vi "face_eye_Detection_test_realTime.vi"() -> ()   [LabVIEW 2010]
uses:
  <vilib>/vision/driver/NI_Vision_Acquisition_Software.lvlib
  <libdir>/resource/objmgr/imaqdx.rc
  <vilib>/vision/NI_Vision_Development_Module.lvlib
  D:/1. DELO FAKS/MOJE/3. Moj OpenCV_dll/face_detection_haar_DLL/build/Release/face_detection_haar_DLL.dll
  <vilib>/Analysis/NI_AALBase.lvlib
  <vilib>/Analysis/baseanly.llb/Mean (DBL).vi
  <vilib>/userdefined/High Color/IMAQdx.ctl
panel:
  out "average detection time [ms]":dbl format="%0.2f"
  out "detected eyes":i32
  out "detected faces":i32
  in  "STOP":bool
  in  "camera":T1="cam0"
  out "processing \ntime [ms]":u32
  out "cascade classifiers loaded?":bool
  out "Image":T2(plugin-control)
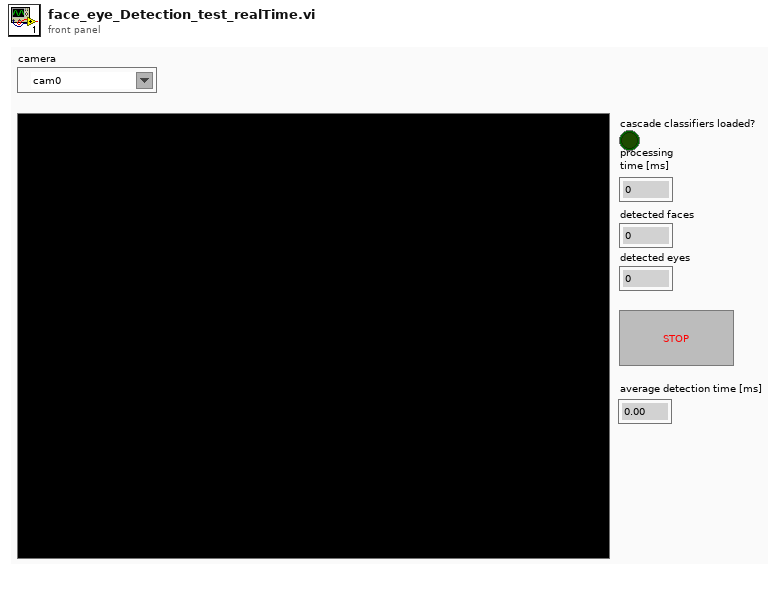
[diagram p1: front panel]
types:
  T1 = typedef "IMAQdx.ctl" = refnum<k21>
  T2 = typedef "IMAQ Image.ctl" = refnum<image>
  T3 = typedef "Image Type" = u32
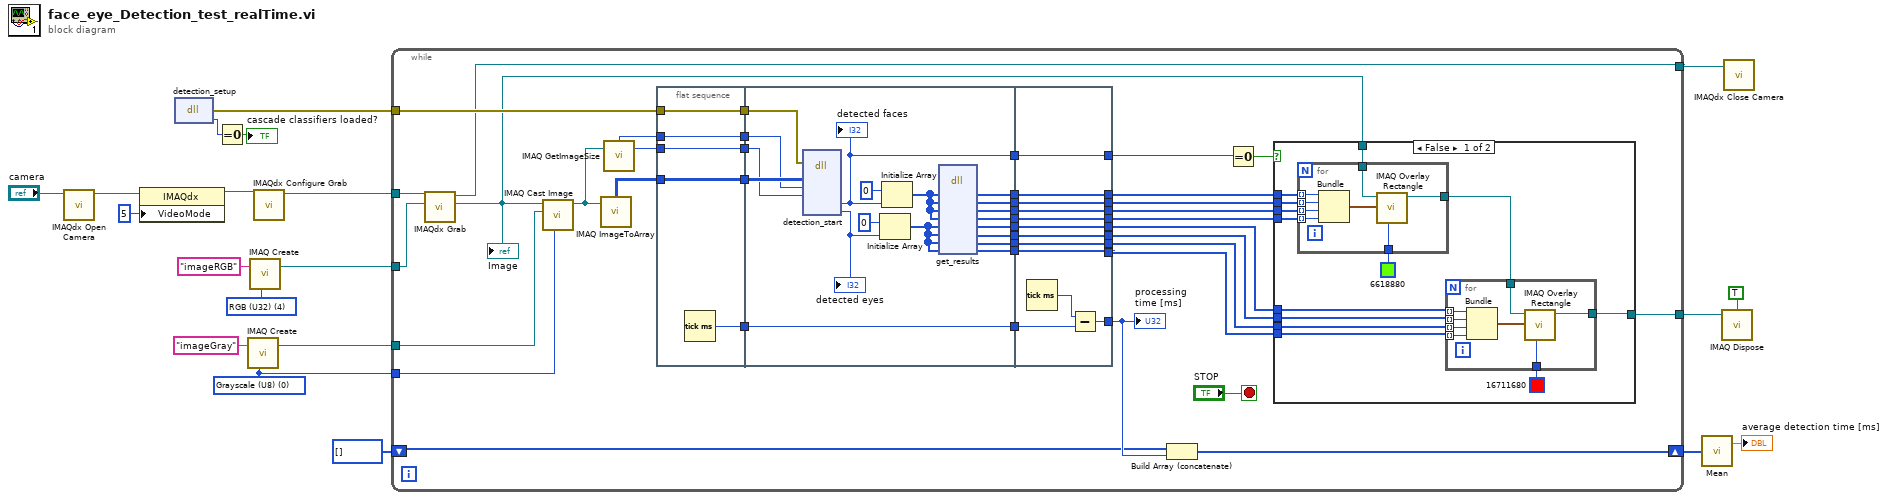
[diagram p0: block diagram]
diagram:
  w6 = T3 0 items=["Grayscale (U8)", "Grayscale (I16)", "Grayscale (SGL)", "Complex (CSG)", "RGB (U32)", "HSL (U32)", "RGB (U64)", "Grayscale (U16)"] ("Image Type")
  w19 = T3 4 items=["Grayscale (U8)", "Grayscale (I16)", "Grayscale (SGL)", "Complex (CSG)", "RGB (U32)", "HSL (U32)", "RGB (U64)", "Grayscale (U16)"] ("Image Type")
  n1 = call <vilib>:"IMAQdx Open Camera.vi"("Session In"="camera") -> ("Session Out"=w14:T1)  [unwired: 9 in, 1 out]
  n2 = property class="IMAQdx"(reference=w14, "VideoMode"=u32 5) -> (reference out=w13:T1)  [unwired: 1 in, 1 out]
  n3 = dll-call lib="D:/1. DELO FAKS/MOJE/3. Moj OpenCV_dll/face_detection_haar_DLL/build/Release/face_detection_haar_DLL.dll" fn="detection_setup"() -> (error out=w18:errorcluster, "return type"=w17:i32)  [unwired: 3 in, 1 out]
  n4 = Equal To 0?(x=w17) -> (x = 0?=→"cascade classifiers loaded?":bool)
  n5 = call "IMAQ Create"("Image Name"="imageGray", "Image Type"=w6) -> ("New Image"=w7:T2)  [unwired: 3 in, 1 out]
  n6 = call "IMAQ Create"("Image Name"="imageRGB", "Image Type"=w19) -> ("New Image"=w10:T2)  [unwired: 3 in, 1 out]
  n7 = call <vilib>:"IMAQdx Configure Grab.vi"("Session In"=w13) -> ("Session Out"=w11:T1)  [unwired: 9 in, 1 out]
  n8 = while {
    tunnel: w18 -> [w51]
    tunnel: w11 -> [w42]
    tunnel: w10 -> [w41]
    tunnel: [w40] -> w9
    tunnel: w7 -> [w38]
    tunnel: w6 -> [w37]
    tunnel: [w24] -> w4
    shift-right: [w22] -> w2
    shift-left: u32[] [] -> [w21]
    stop <- "STOP" stop-if-true
    n9 = call <vilib>:"IMAQdx Grab.vi"("Image In"=w41, "Session In"=w42) -> ("Image Out"=w35:T2, "Session Out"=w40:T1)  [unwired: 6 in, 2 out]
    "Image" <- w35
    n10 = call "IMAQ Cast Image"("Image Type"=w37, "Image Dst"=w38, "Image Src"=w35) -> ("Image Dst Out"=w39:T2)  [unwired: 7 in, 1 out]
    n11 = call "IMAQ ImageToArray"("Image"=w39) -> ("Image Pixels (U8)"=w46:u8[][])  [unwired: 3 in, 4 out]
    n12 = call "IMAQ GetImageSize"("Image"=w39) -> ("Y Resolution"=w44:i32, "X Resolution"=w45:i32)  [unwired: 3 in, 1 out]
    n13 = flat-sequence {
      tunnel: w51 -> [w96]
      tunnel: [w96] -> w61
      tunnel: [w95] -> w60
      tunnel: w46 -> [w94]
      tunnel: [w94] -> w59
      tunnel: w45 -> [w93]
      tunnel: [w93] -> w58
      tunnel: [w92] -> w57
      tunnel: w44 -> [w92]
      tunnel: w61 -> [w115]
      tunnel: [w112] -> w56
      tunnel: [w111] -> w55
      tunnel: [w110] -> w54
      tunnel: [w109] -> w53
      tunnel: [w108] -> w52
      tunnel: w60 -> [w108]
      tunnel: w59 -> [w107]
      tunnel: w58 -> [w106]
      tunnel: w57 -> [w105]
      tunnel: [w102] -> w34
      tunnel: [w101] -> w33
      tunnel: [w100] -> w32
      tunnel: [w99] -> w31
      tunnel: [w98] -> w30
      tunnel: [w124] -> w47
      tunnel: [w125] -> w48
      tunnel: [w126] -> w49
      tunnel: [w127] -> w50
      tunnel: w56 -> [w127]
      tunnel: w55 -> [w126]
      tunnel: w54 -> [w125]
      tunnel: w53 -> [w124]
      tunnel: w52 -> [w122]
      tunnel: [w121] -> w23
      tunnel: w34 -> [w120]
      tunnel: w33 -> [w119]
      tunnel: w32 -> [w118]
      tunnel: w31 -> [w117]
      tunnel: [w120] -> w28
      tunnel: [w119] -> w27
      tunnel: [w118] -> w26
      tunnel: [w117] -> w25
      tunnel: w30 -> [w116]
      tunnel: [w116] -> w29
      frame #0 {
        n14 = Tick Count (ms)() -> (millisecond timer value=w95:u32)
      }
      frame #1 {
        n15 = dll-call lib="D:/1. DELO FAKS/MOJE/3. Moj OpenCV_dll/face_detection_haar_DLL/build/Release/face_detection_haar_DLL.dll" fn="detection_start"(error in=w115, "imdata"=w107, "cols"=w106, "rows"=w105) -> ("result_size_face"=w98:i32, "result_size_eyes"=w97:i32)  [unwired: 8 in, 2 out]
        "detected faces" <- w98
        "detected eyes" <- w97
        n16 = Initialize Array(0 ("element"), w97) -> (w103:i32[])
        n17 = Initialize Array(0 ("element"), w98) -> (w113:i32[])
        n18 = dll-call lib="D:/1. DELO FAKS/MOJE/3. Moj OpenCV_dll/face_detection_haar_DLL/build/Release/face_detection_haar_DLL.dll" fn="get_results"("x1_face"=w113, "y1_face"=w113, "x2_face"=w113, "y2_face"=w113, "x1_eyes"=w103, "y1_eyes"=w103, "x2_eyes"=w103, "y2_eyes"=w103) -> ("x1_face"=w112:i32[], "y1_face"=w111:i32[], "x2_face"=w110:i32[], "y2_face"=w109:i32[], "x1_eyes"=w102:i32[], "y1_eyes"=w101:i32[], "x2_eyes"=w100:i32[], "y2_eyes"=w99:i32[])  [unwired: 4 in, 2 out]
      }
      frame #2 {
        n19 = Tick Count (ms)() -> (millisecond timer value=w123:u32)
        n20 = Subtract(x=w123, y=w122) -> (x-y=w121:u32)
      }
    }
    n21 = Build Array (concatenate)(w21, w23) -> (w22:u32[])
    n22 = Equal To 0?(x=w29) -> (x = 0?=w36:bool)
    n23 = case shown="False" w36 {
      tunnel: w50 -> [w74 _]
      tunnel: w49 -> [w73 _]
      tunnel: w48 -> [w72 _]
      tunnel: w47 -> [w71 _]
      tunnel: w35 -> [w69 w91]
      tunnel: [w62 w91] -> w24
      tunnel: w28 -> [w68 _]
      tunnel: w27 -> [w67 _]
      tunnel: w26 -> [w66 _]
      tunnel: w25 -> [w65 _]
      frame False {
        n24 = for {
          tunnel: w74 -> [w89] mode=indexing
          tunnel: w73 -> [w88] mode=indexing
          tunnel: w72 -> [w87] mode=indexing
          tunnel: w71 -> [w86] mode=indexing
          tunnel: [w90] -> w63
          tunnel: u32 6618880 ("Color") -> [w84]
          tunnel: w69 -> [w83]
          n25 = Bundle(w89, w88, w87, w86) -> (w85:cluster{i32, i32, i32, i32})  [unwired: 1 in]
          n26 = call "IMAQ Overlay Rectangle"("Color"=w84, "Rectangle"=w85, "Image"=w83) -> ("Image Out"=w90:T2)  [unwired: 7 in, 1 out]
        }
        n27 = for {
          tunnel: w68 -> [w81] mode=indexing
          tunnel: w67 -> [w80] mode=indexing
          tunnel: w66 -> [w79] mode=indexing
          tunnel: w65 -> [w78] mode=indexing
          tunnel: [w82] -> w62
          tunnel: u32 16711680 ("Color") -> [w76]
          tunnel: w63 -> [w75]
          n28 = Bundle(w81, w80, w79, w78) -> (w77:cluster{i32, i32, i32, i32})  [unwired: 1 in]
          n29 = call "IMAQ Overlay Rectangle"("Color"=w76, "Rectangle"=w77, "Image"=w75) -> ("Image Out"=w82:T2)  [unwired: 7 in, 1 out]
        }
      }
      frame True {
      }
    }
    "processing \ntime [ms]" <- w23
  }
  n30 = call-poly <vilib>:"Mean.vi"("X"=w2) -> ("mean"=→"average detection time [ms]":dbl)  [unwired: 1 out]
  n31 = call "IMAQ Dispose"("All Images? (No)"=TRUE, "Image"=w4) -> ()  [unwired: 4 in, 1 out]
  n32 = call <vilib>:"IMAQdx Close Camera.vi"("Session In"=w9) -> ()  [unwired: 10 in, 1 out]
